vi "Data File Processing UI Get Message.vi"(8 "error in":errorcluster, 11 "msg queue in":refnum<queue>) -> (0 "error out":errorcluster, 1 "data":variant, 2 "msg":T1, 3 "msg queue out":refnum<queue>)   [LabVIEW 2011]
uses:
  Data File Processing UI Message Define.ctl
  Data File Processing UI Message Type Define.ctl
panel:
  # "Input Data"
  # "Local Data"
  # "Output Data"
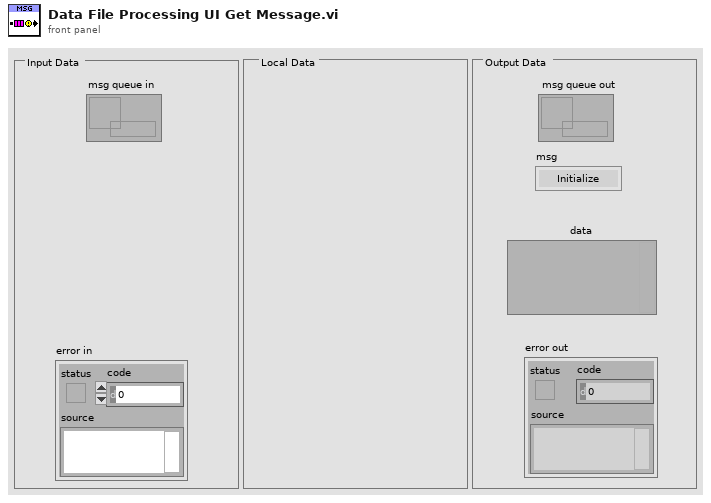
[diagram p1: front panel]
types:
  T1 = typedef "Data File Processing UI Message Type Define.ctl" = enum32{"Initialize", "SleepThread", "ErrorHandler", "NoEvent", "PreExit", "Exit", "----Action----", "OpenFile", "SaveFile", "RedrawGraph", "SelectChannel"}
  T2 = typedef "Data File Processing UI Message Define.ctl" = cluster{"data":variant, "type":T1}
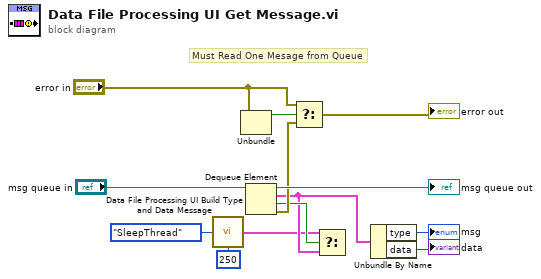
[diagram p0: block diagram]
diagram:
  # "Must Read One Mesage from Queue"
  n1 = call "Data File Processing UI Build Type and Data Message.vi"("type"=Data_File_Processing_UI_Message_Type_Define."SleepThread" ("MsgType"), "data"=u32 250 ("milliseconds to wait")) -> ("msg out"=w1:T2)  [unwired: 13 out]
  n2 = Unbundle("error in") -> ("status"=w11:bool)  [unwired: 2 out]
  n3 = Dequeue Element(queue="msg queue in") -> (queue out=→"msg queue out":refnum<queue>, element=w4:T2, timed out?=w6:bool, error out=w8:errorcluster)  [unwired: 1 in, 1 out]
  n4 = Select(t="error in", s=w11, f=w8) -> (s? t:f=→"error out":errorcluster)
  n5 = Select(t=w1, s=w6, f=w4) -> ()  [unwired: 1 out]
  n6 = Unbundle By Name(w4) -> ("type"=→"msg":T1, "data"=→"data":variant)
